vi "User32.FindWindowA.vi"(5 "lpWindowName":string, 11 "error in (no error)":errorcluster) -> (4 "hwnd":i32, 15 "error out":errorcluster)   [LabVIEW 2021]
uses:
  user32.dll
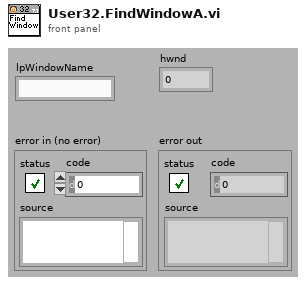
[diagram p1: front panel]
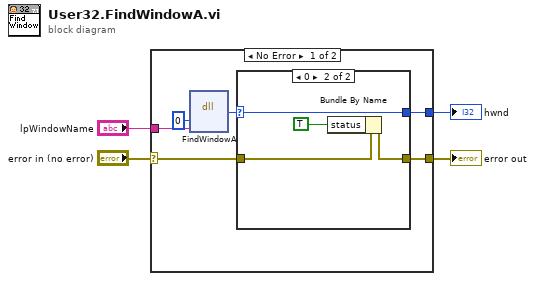
[diagram p0: block diagram]
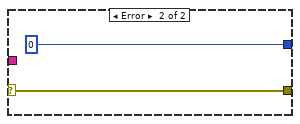
[diagram p3: hidden frame]
diagram:
  n1 = case shown="No Error" "error in (no error)" {
    selector: "error in (no error)" -> [w6 w17]
    tunnel: "lpWindowName" -> [w9 _]
    tunnel: [w7 0] -> w2
    tunnel: [w5 w17] -> w1
    frame No Error {
      n2 = dll-call lib="user32.dll" fn="FindWindowA"("lpClassName"=0, "lpWindowName"=w9) -> (w8:i32)  [unwired: 5 in, 2 out]
      n3 = case shown="0" w8 {
        selector: w8 -> [w12 w16]
        tunnel: [w12 w16] -> w7
        tunnel: w6 -> [w11 w15]
        tunnel: [w11 w14] -> w5
        frame Default {
        }
        frame 0 {
          n4 = Bundle By Name(cluster=w15, "status"=TRUE) -> (w14:errorcluster)
        }
      }
    }
    frame Error {
    }
  }
  "error out" <- w1
  "hwnd" <- w2
